vi "Configure Temperature (RTD).vi"(0 "VISA resource name":refnum<visa-resource-name>, 1 "Enable Offset Compensation (F: Disable)":bool, 5 "Wire Mode (1: 4-Wire)":i16(ring)=1 items=["2-Wire", "4-Wire"], 7 "Unit (0: Celsius)":u16(ring) items=["C", "F", "K"], 9 "Nominal Resistance (100 ohms)":dbl=100.0, 11 "error in (no error)":errorcluster) -> (4 "VISA resource name out":refnum<visa-resource-name>, 15 "error out":errorcluster)   [LabVIEW 2014, in "Agilent 34401.lvlib"]
doc: "Configures the settings for a 2-wire or 4-wire RTD probe.\n\n<B>Note:</B>\n\nThis VI only applies to the 34410/34411 models."
uses:
  <instrlib>/Agilent 34401/Agilent 34401.lvlib
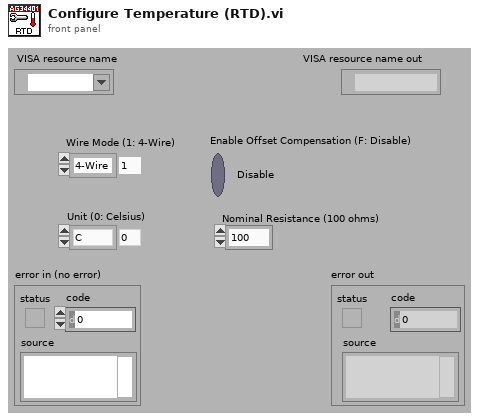
[diagram p1: front panel]
types:
  T1 = typedef "Agilent 34401.lvlib/Extended User Data.ctl" = cluster{"Trigger Source":u16, "Math Storage":u16, "Agilent Model":i32}
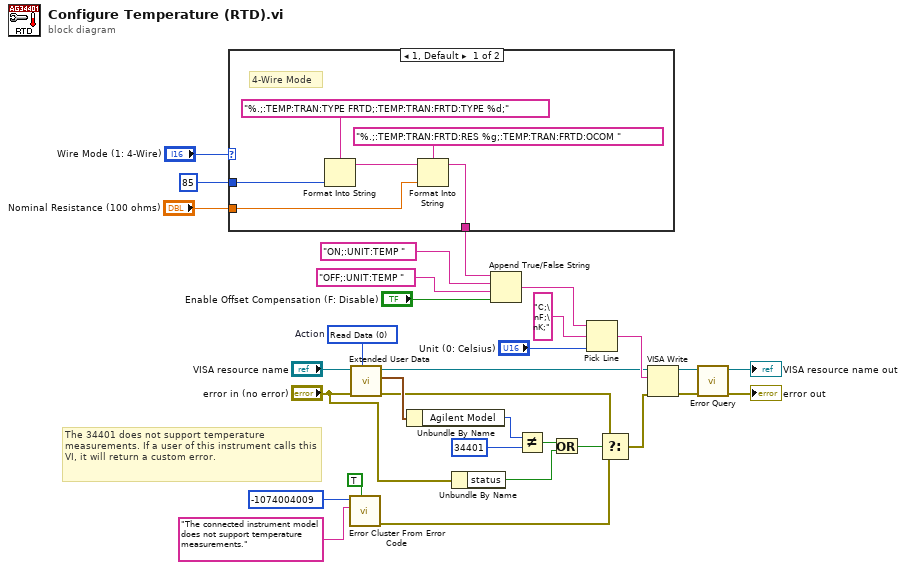
[diagram p0: block diagram]
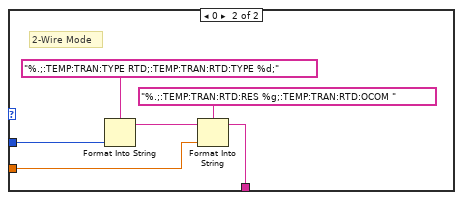
[diagram p2: hidden frame]
diagram:
  w6 = u16 0 items=["Read Data", "Write Data", "Dispose of Data"]  # Action
  # "The 34401 does not support temperature measurements. If a user of this instrument calls this VI, it will return a custom error."
  n1 = case shown="1, Default" "Wire Mode (1: 4-Wire)" {
    tunnel: [w34 w40] -> w21
    tunnel: "Nominal Resistance (100 ohms)" -> [w33 w39]
    tunnel: i16 85 ("input 1") -> [w32 w38]
    frame 1, Default {
      # "4-Wire Mode"
      n2 = Format Into String(format string="%.;:TEMP:TRAN:TYPE FRTD;:TEMP:TRAN:FRTD:TYPE %d;", w32) -> (resulting string=w35:string)  [unwired: 2 in, 1 out]
      n3 = Format Into String(format string="%.;:TEMP:TRAN:FRTD:RES %g;:TEMP:TRAN:FRTD:OCOM ", initial string=w35, w33) -> (resulting string=w34:string)  [unwired: 1 in, 1 out]
    }
    frame 0 {
      # "2-Wire Mode"
      n4 = Format Into String(format string="%.;:TEMP:TRAN:TYPE RTD;:TEMP:TRAN:RTD:TYPE %d;", w38) -> (resulting string=w41:string)  [unwired: 2 in, 1 out]
      n5 = Format Into String(format string="%.;:TEMP:TRAN:RTD:RES %g;:TEMP:TRAN:RTD:OCOM ", initial string=w41, w39) -> (resulting string=w40:string)  [unwired: 1 in, 1 out]
    }
  }
  n6 = call <vilib>:"Error Cluster From Error Code.vi"("show call chain? (False)"=TRUE, "error message (\"\")"="The connected instrument model does not support temperature measurements." ("Source (VI Name)"), "error code (0)"=-1074004009 ("Code")) -> ("error out"=w15:errorcluster)  [unwired: 6 in]
  n7 = call <instrlib>:"Extended User Data.vi"("Action (0: Read Data)"=w6, "Error In (no error)"="error in (no error)", "VISA resource name in"="VISA resource name") -> ("Error Out"=w3:errorcluster, "User Data Out"=w7:T1, "VISA resource name out"=w2:refnum<visa-resource-name>)  [unwired: 6 in]
  n8 = Unbundle By Name(w7) -> ("Agilent Model"=w4:i32)
  n9 = Unbundle By Name("error in (no error)") -> ("status"=w11:bool)
  n10 = Append True/False String(1:"Enable Offset Compensation (F: Disable)", 2:"OFF;:UNIT:TEMP ", 3:"ON;:UNIT:TEMP ", 4:w21) -> (0:w23:string)
  n11 = Not Equal?(x=w4, y=u32 34401 ("x")) -> (x != y?=w13:bool)
  n12 = Or(x=w13, y=w11) -> (x .or. y?=w12:bool)
  n13 = Pick Line(string ("")=w23, multi-line string="C;\nF;\nK;", line index="Unit (0: Celsius)") -> (output string=w16:string)
  n14 = Select(t=w3, s=w12, f=w15) -> (s? t:f=w14:errorcluster)
  n15 = VISA Write(VISA resource name=w2, write buffer=w16, error in (no error)=w14) -> (VISA resource name out=w29:refnum<visa-resource-name>, error out=w28:errorcluster)  [unwired: 1 out]
  n16 = call <instrlib>:"Error Query.vi"("error in (no error)"=w28, "VISA resource name"=w29) -> ("error out"=→"error out":errorcluster, "VISA resource name out"=→"VISA resource name out":refnum<visa-resource-name>)  [unwired: 6 in, 2 out]
